vi "WPI_IMU_ADIS16448_WriteReadRegister.vi"(8 "error in (no error)":errorcluster, 9 "Data":u16=2049, 10 "ADIS16448 Register":T1=54 items=["SMPL_PRD"=54, "SENS_AVG"=56, "MSC_CTRL"=52, "ERROR_FLAGS"=60, "TEMP"=44, "BARO"=40, "Z_MAG"=36, "Y_MAG"=32, "X_MAG"=28, "Z_ACCEL"=24, "Y_ACCEL"=20, "X_ACCEL"=16, "Z_GYRO"=12, "Y_GYRO"=8, "X_GYRO"=4, "PID"=86], 11 "SPIDevRef in":T2) -> (0 "error out":errorcluster, 1 "Write OK?":bool, 2 "Register Value":u16, 3 "SPIDevRef out":T2)   [LabVIEW 2015, in "Apple Pi Gyro Library.lvlib" / "FRC_ADIS16448_IMU.lvlib"]
uses:
  FRC_ADIS16448_IMU.lvlib
  <vilib>/Rock Robotics/WPI/SPI/WPI_SPIDevRef.ctl
  <vilib>/Rock Robotics/SystemInterfaces/spilib/spi_bus.ctl
  WPI_IMU_ADIS16448_Registers.ctl
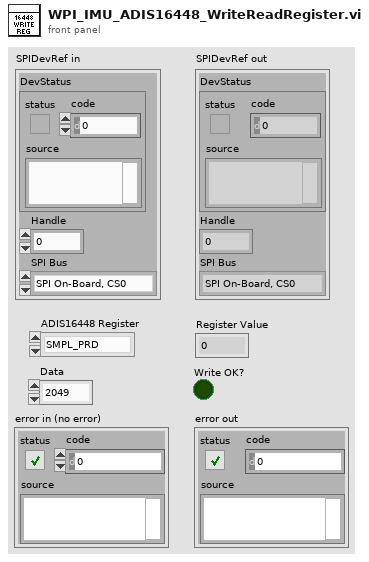
[diagram p1: front panel]
types:
  T1 = typedef "Apple Pi Gyro Library.lvlib/FRC_ADIS16448_IMU.lvlib/WPI_IMU_ADIS16448_Registers.ctl" = u8
  T2 = typedef "WPI_SPIDevRef.ctl" = cluster{"DevStatus":errorcluster, "Handle":i32, "SPI Bus":T3}
  T3 = typedef "spi_bus.ctl" = enum16{"SPI On-Board, CS0", "SPI On-Board, CS1", "SPI On-Board, CS2", "SPI On-Board, CS3", "SPI MXP", "Invalid"}
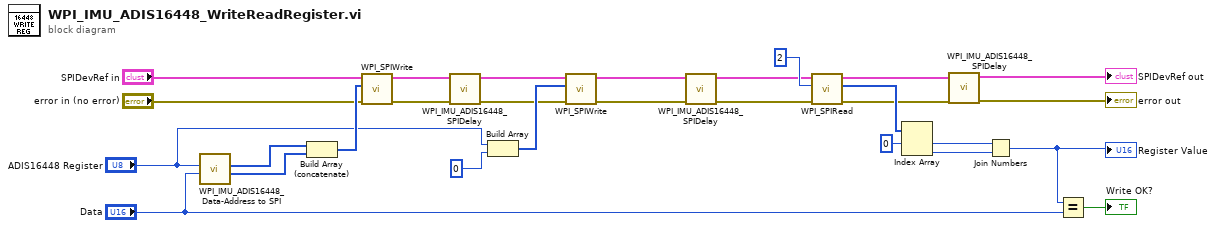
[diagram p0: block diagram]
diagram:
  n1 = call "WPI_IMU_ADIS16448_Data-Address to SPI.vi"("Data"="Data", "Address"="ADIS16448 Register") -> ("Low Word"=w23:u8[], "High Word"=w24:u8[])  [unwired: 8 in]
  n2 = Build Array (concatenate)(w24, w23) -> (w25:u8[])
  n3 = call <vilib>:"WPI_SPIWrite.vi"("error in (no error)"="error in (no error)", "Data To Send"=w25, "SPIDevRef"="SPIDevRef in") -> ("error out"=w9:errorcluster, "SPIDevRef"=w10:T2)  [unwired: 7 out]
  n4 = call "WPI_IMU_ADIS16448_SPIDelay.vi"("error in"=w9, "SPIDevRef in"=w10) -> ("error out"=w11:errorcluster, "SPIDevRef out"=w12:T2)  [unwired: 8 in]
  n5 = Build Array("ADIS16448 Register", 0) -> (w22:i32[])
  n6 = call <vilib>:"WPI_SPIWrite.vi"("error in (no error)"=w11, "Data To Send"=w22, "SPIDevRef"=w12) -> ("error out"=w7:errorcluster, "SPIDevRef"=w8:T2)  [unwired: 7 out]
  n7 = call "WPI_IMU_ADIS16448_SPIDelay.vi"("error in"=w7, "SPIDevRef in"=w8) -> ("error out"=w6:errorcluster, "SPIDevRef out"=w5:T2)  [unwired: 8 in]
  n8 = call <vilib>:"WPI_SPIRead.vi"("error in (no error)"=w6, "Num to Read"=2, "SPIDevRef"=w5) -> ("error out"=w3:errorcluster, "Received Data"=w26:u8[], "SPIDevRef"=w4:T2)  [unwired: 6 in]
  n9 = Index Array(array=w26, index #1=0 ("index")) -> (element #1=w19:u8, element #2=w18:u8)  [unwired: 1 in]
  n10 = call "WPI_IMU_ADIS16448_SPIDelay.vi"("error in"=w3, "SPIDevRef in"=w4) -> ("error out"=→"error out":errorcluster, "SPIDevRef out"=→"SPIDevRef out":T2)  [unwired: 8 in]
  n11 = Join Numbers(hi=w19, lo=w18) -> ((hi.lo)=w17:u16)
  "Register Value" <- w17
  n12 = Equal?(x=w17, y="Data") -> (x = y?=→"Write OK?":bool)
